vi "Write HSMS Class.vi"(8 "error in (no error)":errorcluster, 10 "HSMS Class":refnum<class "HSMS Class.lvclass">, 11 "Scenarios Class in":refnum<class "Scenarios Class.lvclass">) -> (0 "error out":errorcluster, 3 "Scenarios Class out":refnum<class "Scenarios Class.lvclass">)   [LabVIEW 2020, in "SECS Scenarios.lvlib" / "Scenarios Class.lvclass"]
uses:
  Scenarios Class.lvclass
  SECS Communication/HSMS Class/HSMS Class.lvclass
  Scenarios Class.lvclass/Scenarios Class.ctl
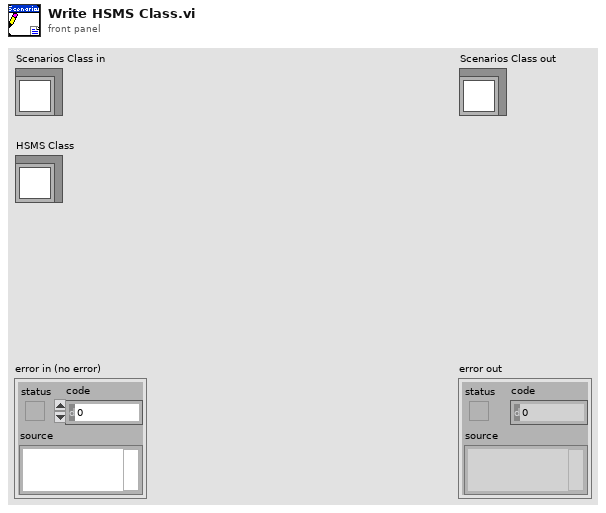
[diagram p1: front panel]
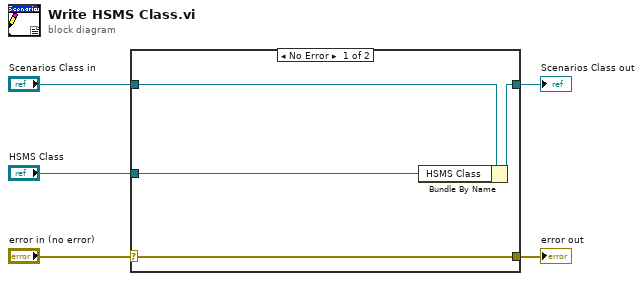
[diagram p0: block diagram]
diagram:
  n1 = case shown="No Error" "error in (no error)" {
    selector: "error in (no error)" -> [w9 w10]
    tunnel: [w9 w10] -> w4
    tunnel: [w7 w11] -> w2
    tunnel: "Scenarios Class in" -> [w8 w11]
    tunnel: "HSMS Class" -> [w6 _]
    frame No Error {
      n2 = Bundle By Name(cluster=w8, "HSMS Class"=w6) -> (w7:refnum<class "Scenarios Class.lvclass">)
    }
    frame Error {
    }
  }
  "error out" <- w4
  "Scenarios Class out" <- w2
